vi "Pulse Generator.vi"(10 "Input Valid":bool, 11 "Data":bool) -> (2 "Ready For Input":bool, 3 "Pulse Output":bool)   [LabVIEW 2021, in "Neopixel - FPGA.lvclass"]
uses:
  Neopixel - FPGA.lvclass
  Controls/Pulse Generation State.ctl
  Neopixel - FPGA.lvclass/Neopixel - FPGA.ctl
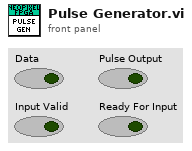
[diagram p1: front panel]
types:
  T1 = typedef "Neopixel - FPGA.lvclass/Pulse Generation State.ctl" = enum16{"High", "Low", "Idle"}
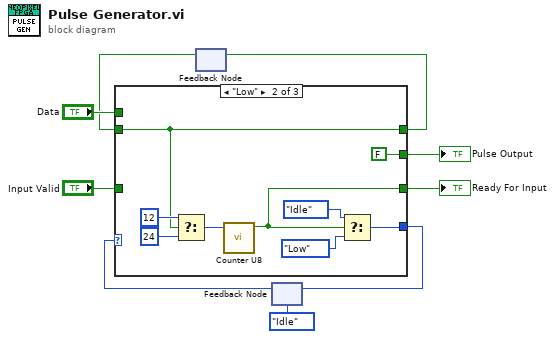
[diagram p0: block diagram]
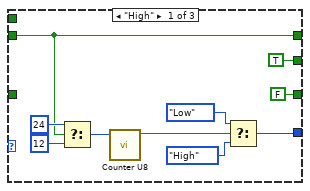
[diagram p2: hidden frame]
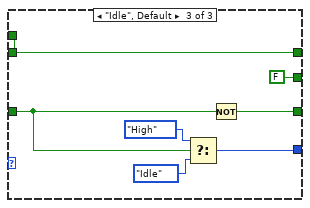
[diagram p3: hidden frame]
diagram:
  n1 = feedback #1() -> (w2:bool)  [unwired: 1 in]
  n2 = feedback #2(Pulse_Generation_State."Idle") -> (w6:T1)
  n3 = case shown="\"Low\"" w6 {
    tunnel: [TRUE FALSE FALSE] -> w8
    tunnel: [w15 w27 w32] -> w5
    tunnel: [FALSE ("Value Reached") w24 w30] -> w9
    tunnel: "Data" -> [_ _ w35]
    tunnel: [w10 w20 w35] -> w3
    tunnel: w2 -> [w10 w20 _]
    tunnel: "Input Valid" -> [_ _ w31]
    frame "High" {
      n4 = Select(t=u8 24 ("High True"), s=w10, f=u8 12 ("High False")) -> (s? t:f=w11:u8)
      n5 = call "Counter U8.vi"("Count To"=w11) -> ("Value Reached"=w18:bool)  [unwired: 9 in, 1 out]
      n6 = Select(t=Pulse_Generation_State."Low", s=w18, f=Pulse_Generation_State."High") -> (s? t:f=w15:T1)
    }
    frame "Low" {
      n7 = Select(t=u8 12 ("High True"), s=w20, f=u8 24 ("High False")) -> (s? t:f=w21:u8)
      n8 = call "Counter U8.vi"("Count To"=w21) -> ("Value Reached"=w24:bool)  [unwired: 9 in, 1 out]
      n9 = Select(t=Pulse_Generation_State."Idle", s=w24, f=Pulse_Generation_State."Low") -> (s? t:f=w27:T1)
    }
    frame "Idle", Default {
      n10 = Select(t=Pulse_Generation_State."High", s=w31, f=Pulse_Generation_State."Idle") -> (s? t:f=w32:T1)
      n11 = Not(x=w31) -> (.not. x?=w30:bool)
    }
  }
  "Ready For Input" <- w9
  "Pulse Output" <- w8
  n12 = feedback-in #1(w3) -> ()
  n13 = feedback-in #2(w5) -> ()
